vi "Verificar Estado Cola.vi"(7 "Estado Timer In":T1(ring)=enum."Get Time", 10 "Cola":refnum<queue>, 11 "Cola GUI":refnum<queue>) -> (0 "error out":errorcluster, 1 "# elem in queue":i32(slide) scale=0.0..200.0, 3 "Queue out":refnum<queue>, 5 "Estado Timer Out":T1(ring)=enum."Get Time")   [LabVIEW 2018, in "Support VIs.lvlib"]
uses:
  QMH_Topside/Support VIs/Support VIs.lvlib
  Message Cluster.ctl
  Enqueue Message (Single).vi
  Message Queue.lvlib
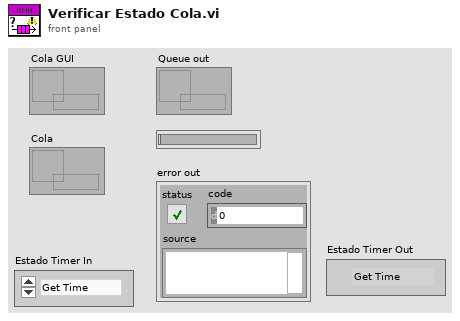
[diagram p1: front panel]
types:
  T1 = enum16{"Start Timer", "Get Time", "Pause", "Unpause"}
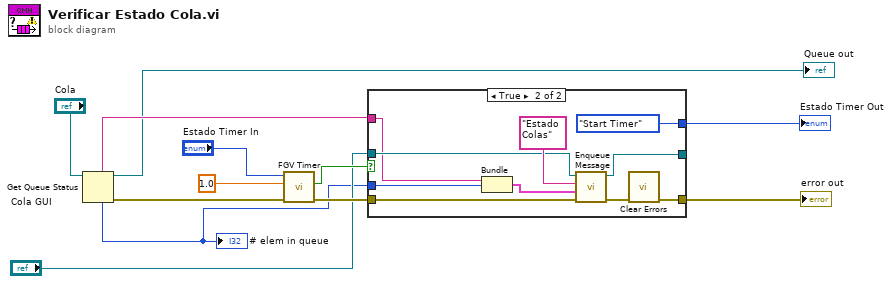
[diagram p0: block diagram]
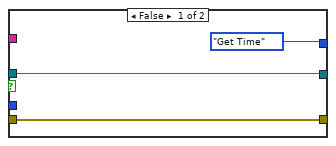
[diagram p2: hidden frame]
diagram:
  n1 = Get Queue Status(queue="Cola") -> (queue out=→"Queue out":refnum<queue>, queue name=w3:string, error out=w2:errorcluster, # elements in queue=w6:i32)  [unwired: 2 in, 4 out]
  "# elem in queue" <- w6
  n2 = call "FGV Timer.vi"("error in (no error)"=w2, "Target Time"=1.0, "Enum"="Estado Timer In") -> ("error out"=w10:errorcluster, "Time Elapsed?"=w11:bool)  [unwired: 5 in, 2 out]
  n3 = case shown="True" w11 {
    tunnel: [w14 w22] -> w4
    tunnel: "Cola GUI" -> [w15 w24]
    tunnel: [w15 w21] -> _
    tunnel: w10 -> [w14 w20]
    tunnel: w6 -> [_ w19]
    tunnel: w3 -> [_ w18]
    tunnel: [T1."Get Time" ("Enum") T1."Start Timer" ("Enum")] -> w5
    frame False {
    }
    frame True {
      n4 = Bundle(w18, "# elements in queue"=w19) -> (w17:cluster{string, "# elements in queue":i32})  [unwired: 1 in]
      n5 = call-poly "Enqueue Message.vi"("error in (no error)"=w20, "Message Data"=w17, "Message"="Estado Colas", "Message Queue"=w24) -> ("error out"=w23:errorcluster, "dup Message Queue"=w21:refnum<queue>)  [unwired: 6 in]
      n6 = call <vilib>:"Clear Errors.vi"("error in (no error)"=w23) -> ("error out"=w22:errorcluster)  [unwired: 5 in, 1 out]
    }
  }
  "error out" <- w4
  "Estado Timer Out" <- w5
